vi "Tree Map to XML Recursive.vi"(6 "Preserve Insertion Order? (F)":bool, 7 "Indent":i32, 10 "Path Set":set{string}(c389), 11 "Tree Map In":T1) -> (3 "XML Lines":string[](array[string]), 4 "Path Invalid":bool)   [LabVIEW 2020, in "Tree Map.lvlib"]
doc: "<b>Author:</b> Piotr Kruczkowski <PrimaryKey>\n<b>License:</b> NewBSD\n\nCopyright (c) 2019, National Instruments\nAll rights reserved.\n\nRedistribution and use in source and binary forms, with or without\nmodification, are permitted provided that the following conditions are met:\n1. Redistributions of source code must retain the above copyright\n notice, this list of conditions and the following disclaimer.\n2. Redistributions in binary form must reproduce the above copyright\n notice, this list of conditions and the following disclaimer in the\n documentation and/or other materials provided with the distribution.\n3. Neither the name of National Instruments nor the\n names of its contributors may be used to endorse or promote products\n derived from this software without specific prior written permission.\n\nTHIS SOFTWARE IS PROVIDED BY National Instruments ''AS IS'' AND ANY\nEXPRESS OR IMPLIED WARRANTIES, INCLUDING, BUT NOT LIMITED TO, THE IMPLIED\nWARRANTIES OF MERCHANTABILITY AND FITNESS FOR A PARTICULAR PURPOSE ARE\nDISCLAIMED. IN NO EVENT SHALL National Instruments BE LIABLE FOR ANY\nDIRECT, INDIRECT, INCIDENTAL, SPECIAL, EXEMPLARY, OR CONSEQUENTIAL DAMAGES\n(INCLUDING, BUT NOT LIMITED TO, PROCUREMENT OF SUBSTITUTE GOODS OR SERVICES;\nLOSS OF USE, DATA, OR PROFITS; OR BUSINESS INTERRUPTION) HOWEVER CAUSED AND\nON ANY THEORY OF LIABILITY, WHETHER IN CONTRACT, STRICT LIABILITY, OR TORT\n(INCLUDING NEGLIGENCE OR OTHERWISE) ARISING IN ANY WAY OUT OF THE USE OF THIS\nSOFTWARE, EVEN IF ADVISED OF THE POSSIBILITY OF SUCH DAMAGE."
uses:
  Tree Map.lvlib
  Tree Map Data.ctl
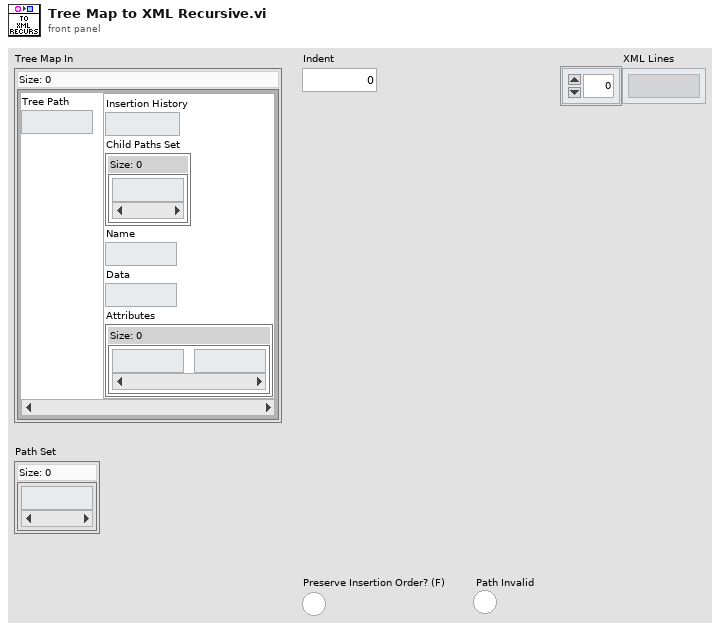
[diagram p1: front panel]
types:
  T1 = typedef "Tree Map.lvlib/Tree Map Data.ctl" = map{string, cluster{"Insertion History":i32, "Child Paths Set":set{string}, "Name":string, "Data":string, "Attributes":map{string, string}}}
  T2 = cluster{"Insertion History":i32, "Child Paths Set":set{string}, "Name":string, "Data":string, "Attributes":map{string, string}}
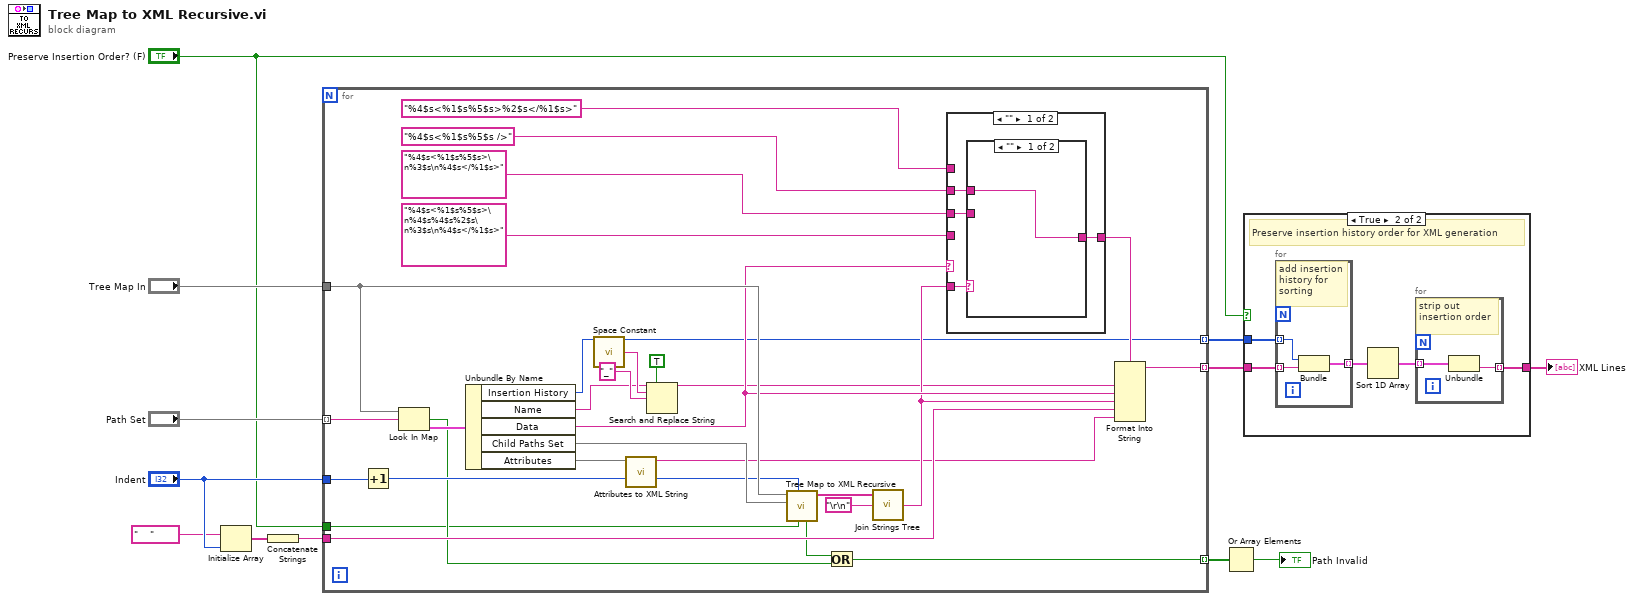
[diagram p0: block diagram]
diagram:
  n1 = Initialize Array("    ", "Indent") -> (w10:string[])
  n2 = Concatenate Strings(w10) -> (w11:string)
  n3 = for {
    tunnel: w11 -> [w35]
    tunnel: "Indent" -> [w41]
    tunnel: "Path Set" -> [w33] mode=indexing
    tunnel: "Tree Map In" -> [w38]
    tunnel: [w20] -> w7 mode=indexing
    tunnel: "Preserve Insertion Order? (F)" -> [w15]
    tunnel: [w14] -> w3 mode=indexing
    tunnel: [w13] -> w2 mode=indexing
    n4 = Increment(x=w41) -> (x+1=w34:i32)
    n5 = Look In Map(map=w38, key=w33) -> (key not found?=w21:bool, value=w40:T2)  [unwired: 1 in]
    n6 = Unbundle By Name(w40) -> ("Insertion History"=w13:i32, "Name"=w16:string, "Data"=w32:string, "Child Paths Set"=w39:set{string}, "Attributes"=w18:map{string, string})
    n7 = call <vilib>:"Space Constant.vi"() -> ("String"=w26:string)
    n8 = call "Attributes to XML String.vi"("Attributes"=w18) -> ("XML String"=w17:string)  [unwired: 10 in]
    n9 = Search and Replace String(replace all?=TRUE ("replace all? (F)"), input string=w16, search string=w26, replace string="_") -> (result string=w23:string)  [unwired: 4 in, 3 out]
    n10 = call "Tree Map to XML Recursive.vi"("Preserve Insertion Order? (F)"=w15, "Indent"=w34, "Path Set"=w39, "Tree Map In"=w38) -> ("XML Lines"=w37:string[], "Path Invalid"=w22:bool)  [unwired: 6 in]
    n11 = Or(x=w22, y=w21) -> (x .or. y?=w20:bool)
    n12 = call "Join Strings Tree.vi"("Separator"="\r\n", "Strings In"=w37) -> ("String"=w31:string)  [unwired: 1 in]
    n13 = case shown="\"\"" w32 {
      tunnel: w31 -> [w45 w51]
      tunnel: "%4$s<%1$s%5$s>%2$s</%1$s>" ("format string") -> [_ w50]
      tunnel: "%4$s<%1$s%5$s>\n%4$s%4$s%2$s\n%3$s\n%4$s</%1$s>" ("format string") -> [_ w49]
      tunnel: [w44 w48] -> w30
      tunnel: "%4$s<%1$s%5$s>\n%3$s\n%4$s</%1$s>" ("format string") -> [w42 _]
      tunnel: "%4$s<%1$s%5$s />" ("format string") -> [w43 _]
      frame "" {
        n14 = case shown="\"\"" w45 {
          tunnel: [w46 w47] -> w44
          tunnel: w43 -> [w46 _]
          tunnel: w42 -> [_ w47]
          frame "" {
          }
          frame Default {
          }
        }
      }
      frame Default {
        n15 = case shown="\"\"" w51 {
          tunnel: w50 -> [w52 _]
          tunnel: w49 -> [_ w53]
          tunnel: [w52 w53] -> w48
          frame "" {
          }
          frame Default {
          }
        }
      }
    }
    n16 = Format Into String(format string=w30, w23, w32, w31, w35, w17) -> (resulting string=w14:string)  [unwired: 2 in, 1 out]
  }
  n17 = Or Array Elements(Boolean array=w7) -> (logical OR=→"Path Invalid":bool)
  n18 = case shown="True" "Preserve Insertion Order? (F)" {
    tunnel: [w54 w58] -> w4
    tunnel: w3 -> [w54 w57]
    tunnel: w2 -> [_ w56]
    frame False {
      # "Do not preserve insertion order for XML generation"
    }
    frame True {
      # "Preserve insertion history order for XML generation"
      n19 = for {
        tunnel: w56 -> [w62] mode=indexing
        tunnel: w57 -> [w61] mode=indexing
        tunnel: [w60] -> w55 mode=indexing
        # "add insertion history for sorting"
        n20 = Bundle("Insertion History"=w62, w61) -> (w60:cluster{"Insertion History":i32, string})  [unwired: 1 in]
      }
      n21 = Sort 1D Array(array=w55) -> (sorted array=w59:cluster{"Insertion History":i32, string}[])
      n22 = for {
        tunnel: w59 -> [w64] mode=indexing
        tunnel: [w63] -> w58 mode=indexing
        # "strip out insertion order"
        n23 = Unbundle(w64) -> (w63:string)  [unwired: 1 out]
      }
    }
  }
  "XML Lines" <- w4
